vi "IVI DC Power Supply Main Page.vi"(8 "error in (no error)":errorcluster, 11 "Node Ptr":T1 format="%.0x") -> (0 "error out":errorcluster)   [LabVIEW 2011, in "IVI DC Power Supply Custom Device.lvlib"]
uses:
  IVI DC Power Supply Custom Device.lvlib
  <vilib>/NI Veristand/Custom Device API/Custom Device Item Ref.ctl
  Global.vi
  <vilib>/NI Veristand/Custom Device API/Get Item Property (String).vi
  <vilib>/NI Veristand/Custom Device API/Get Item Property (Double).vi
  <vilib>/NI Veristand/Custom Device API/Set Item Property (String).vi
  <vilib>/NI Veristand/Custom Device API/Set Item Property (Double).vi
  <vilib>/NI Veristand/Custom Device API/Custom Device API.lvlib
panel:
  in  "Desired Loop Rate (Hz)":dbl=0.5
  in  "Logical Name in MAX":string
  in  "Header":cluster{"Section Name":string}={"Section Name"="IVI DC Power Supply Settings"}
  in  "Description":string
  in  "IVI DC Power Supply Name":string
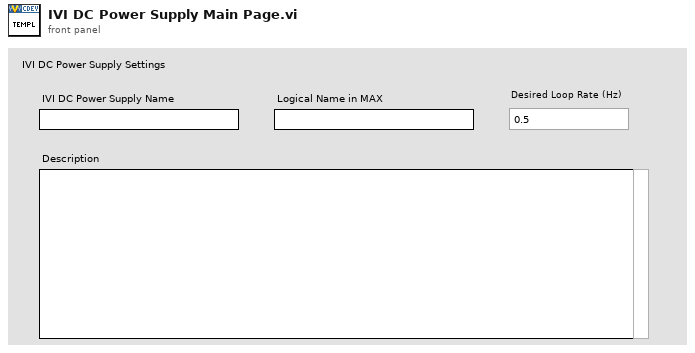
[diagram p1: front panel]
types:
  T1 = typedef "Custom Device API.lvlib/Custom Device Item Ref.ctl" = u64
  T2 = typedef "Custom Device API.lvlib/Custom Device Item Info.ctl" = cluster{"Name":string, "Is Channel":bool, "GUID":string}
  T3 = typedef "Custom Device API.lvlib/Custom Device Commands.ctl" = enum16{"Default", "Item renamed", "Shutdown", "Dynamic button pressed"}
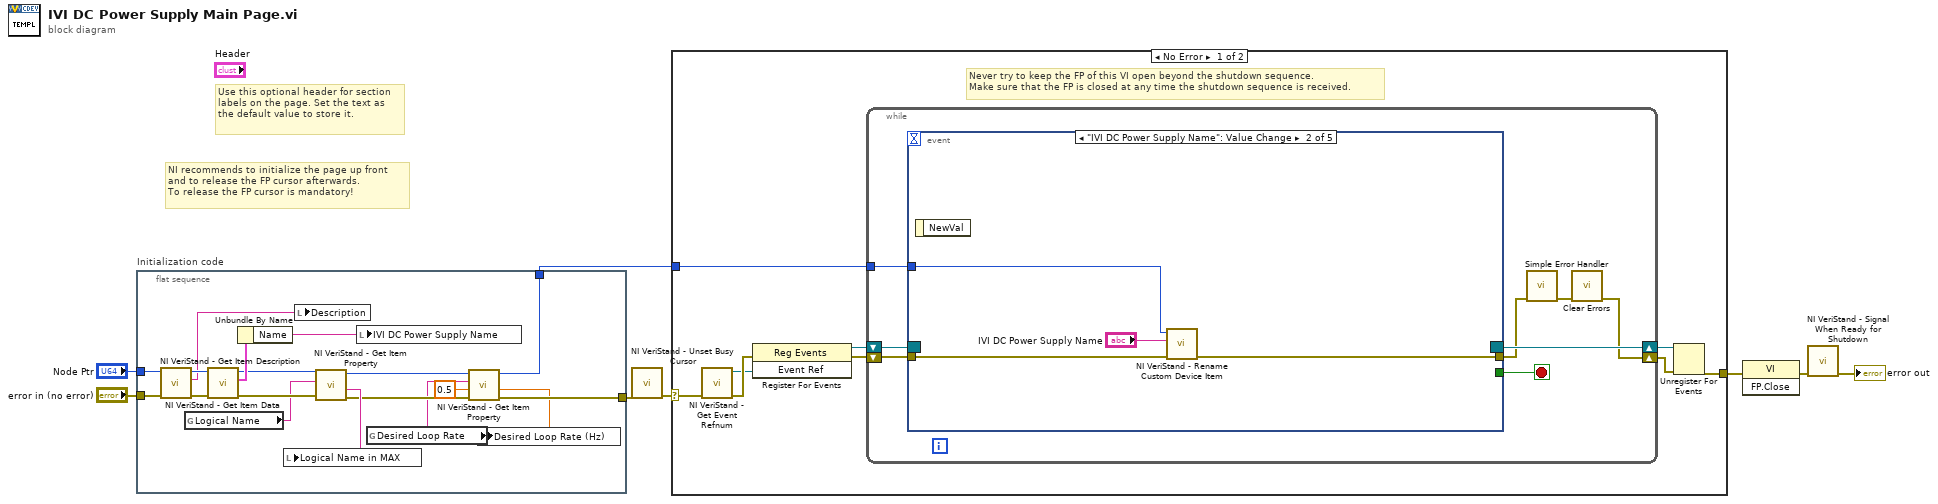
[diagram p0: block diagram]
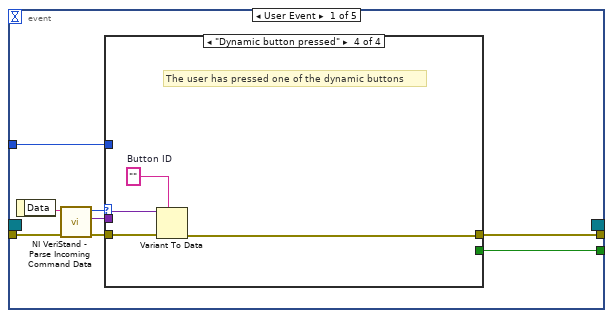
[diagram p2: hidden frame]
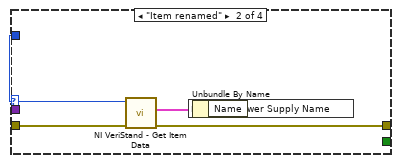
[diagram p4: hidden frame]
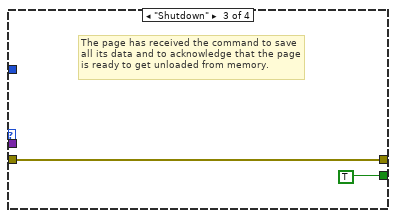
[diagram p5: hidden frame]
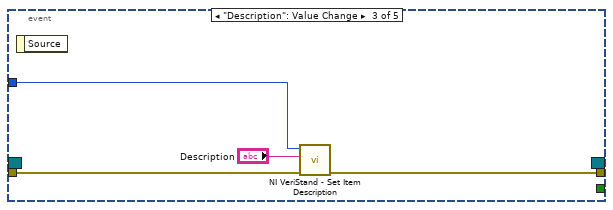
[diagram p6: hidden frame]
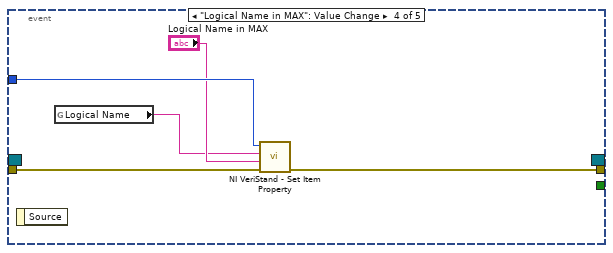
[diagram p7: hidden frame]
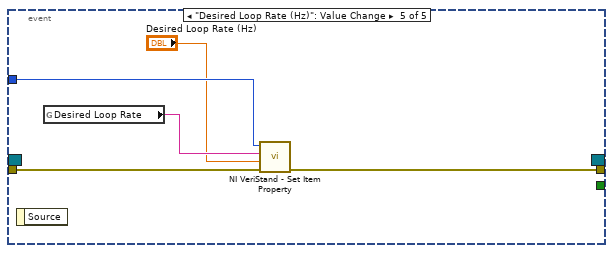
[diagram p8: hidden frame]
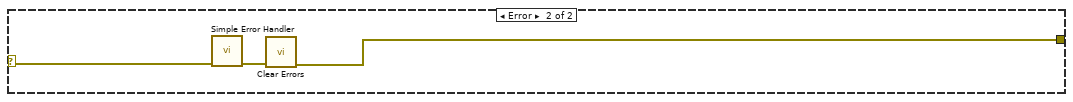
[diagram p9: hidden frame]
diagram:
  # "Use this optional header for section labels on the page. Set the text as the default value to store it."
  # "NI recommends to initialize the page up front\nand to release the FP cursor afterwards.\nTo release the FP cursor is mandatory!"
  n1 = flat-sequence "Initialization code" {
    tunnel: "error in (no error)" -> [w25]
    tunnel: "Node Ptr" -> [w24]
    tunnel: [w13] -> w2
    tunnel: [w12] -> w1
    frame #0 {
      n2 = call <vilib>:"NI VeriStand - Get Item Description.vi"("error in (no error)"=w25, "Item Ref in"=w24) -> ("error out"=w22:errorcluster, "Description"=w23:string, "Item Ref out"=w26:T1)  [unwired: 7 out]
      n3 = global read "Global.vi" "Logical Name"() -> (w17:string)
      n4 = call <vilib>:"NI VeriStand - Get Item Data.vi"("error in (no error)"=w22, "Item Ref in"=w26) -> ("error out"=w18:errorcluster, "Item Info"=w21:T2, "Item Ref out"=w19:T1)  [unwired: 7 out]
      n5 = Unbundle By Name(w21) -> ("Name"=w20:string)
      n6 = local write "Description"(w23) -> ()
      n7 = call-poly <vilib>:"NI VeriStand - Get Item Property.vi"("error in (no error)"=w18, "Property Name"=w17, "Item Ref in"=w19) -> ("error out"=w15:errorcluster, "Value"=w16:string, "Item Ref out"=w14:T1)  [unwired: 5 in, 1 out]
      n8 = local write "Logical Name in MAX"(w16) -> ()
      n9 = local write "IVI DC Power Supply Name"(w20) -> ()
      n10 = global read "Global.vi" "Desired Loop Rate"() -> (w11:string)
      n11 = call-poly <vilib>:"NI VeriStand - Get Item Property.vi"("error in (no error)"=w15, "Default Value"=0.5, "Property Name"=w11, "Item Ref in"=w14) -> ("error out"=w12:errorcluster, "Value"=w10:dbl, "Item Ref out"=w13:T1)  [unwired: 4 in, 1 out]
      n12 = local write "Desired Loop Rate (Hz)"(w10) -> ()
    }
  }
  n13 = call <vilib>:"NI VeriStand - Unset Busy Cursor.vi"("error in (no error)"=w1) -> ("error out"=w4:errorcluster)  [unwired: 10 out]
  n14 = case shown="No Error" w4 {
    selector: w4 -> [w27 w84]
    tunnel: [w32 w82] -> w8
    tunnel: w2 -> [w28 _]
    frame No Error {
      # "Never try to keep the FP of this VI open beyond the shutdown sequence.\nMake sure that the FP is closed at any time the shutdown sequence is received."
      n15 = call <vilib>:"NI VeriStand - Get Event Refnum.vi"("error in (no error)"=w27) -> ("error out"=w35:errorcluster, "Event Ref"=w31:refnum<user-event>)  [unwired: 9 out]
      n16 = register-events(error in=w35, w31) -> (reference out=w29:refnum<event-registration>, error out=w30:errorcluster)  [unwired: 1 in]
      n17 = while {
        tunnel: w28 -> [w39]
        shift-right: [w36] -> w33
        shift-left: w30 -> [w42]
        shift-right: [w43] -> w34
        shift-left: w29 -> [w41]
        stop <- w40 stop-if-true
        n18 = event shown="[1] \"IVI DC Power Supply Name\": Value Change" {
          selector: w41 -> [_ _ _ _ _]
          dyn-events: [_ _ _ _ _] -> w43
          timeout: _ -> [_ _ _ _ _]
          tunnel: w42 -> [w51 w67 w70 w76 w81]
          tunnel: [w47 _ _ _ _] -> w40
          tunnel: [w46 w66 w69 w75 w80] -> w38
          tunnel: w39 -> [w45 w65 w71 w74 w79]
          event User Event {
            n19 = event-data() -> ("Data"=w50:string)  [unwired: 1 out]
            n20 = call <vilib>:"NI VeriStand - Parse Incoming Command Data.vi"("error in (no error)"=w51, "Incoming data"=w50) -> ("error out"=w49:errorcluster, "Outgoing data"=w44:variant, "Action"=w48:T3)  [unwired: 7 out]
            n21 = case shown="\"Dynamic button pressed\"" w48 {
              tunnel: w49 -> [w52 w57 w58 w63]
              tunnel: [_ _ TRUE _] -> w47
              tunnel: [w52 w54 w58 w60] -> w46
              tunnel: w45 -> [_ w56 _ _]
              tunnel: w44 -> [_ _ _ w62]
              frame "Default", Default {
              }
              frame "Item renamed" {
                n22 = call <vilib>:"NI VeriStand - Get Item Data.vi"("error in (no error)"=w57, "Item Ref in"=w56) -> ("error out"=w54:errorcluster, "Item Info"=w55:T2)  [unwired: 8 out]
                n23 = Unbundle By Name(w55) -> ("Name"=w53:string)
                n24 = local write "IVI DC Power Supply Name"(w53) -> ()
              }
              frame "Shutdown" {
                # "The page has received the command to save all its data and to acknowledge that the page is ready to get unloaded from memory."
              }
              frame "Dynamic button pressed" {
                w61 = ""  # Button ID
                # "The user has pressed one of the dynamic buttons"
                n25 = Variant To Data(error in=w63, type=w61, Variant=w62) -> (error out=w60:errorcluster)  [unwired: 1 out]
              }
            }
          }
          event "IVI DC Power Supply Name": Value Change {
            n26 = event-data() -> ()  [unwired: 2 out]
            n27 = call <vilib>:"NI VeriStand - Rename Custom Device Item.vi"("error in (no error)"=w67, "New Name"="IVI DC Power Supply Name", "Item Ref in"=w65) -> ("error out"=w66:errorcluster)  [unwired: 8 out]
          }
          event "Description": Value Change {
            n28 = event-data() -> ()  [unwired: 2 out]
            n29 = call <vilib>:"NI VeriStand - Set Item Description.vi"("error in (no error)"=w70, "Description"="Description", "Item Ref in"=w71) -> ("error out"=w69:errorcluster)  [unwired: 8 out]
          }
          event "Logical Name in MAX": Value Change {
            n30 = event-data() -> ()  [unwired: 2 out]
            n31 = global read "Global.vi" "Logical Name"() -> (w72:string)
            n32 = call-poly <vilib>:"NI VeriStand - Set Item Property.vi"("error in (no error)"=w76, "Value"="Logical Name in MAX", "Property Name"=w72, "Item Ref in"=w74) -> ("error out"=w75:errorcluster)  [unwired: 5 in, 2 out]
          }
          event "Desired Loop Rate (Hz)": Value Change {
            n33 = event-data() -> ()  [unwired: 2 out]
            n34 = global read "Global.vi" "Desired Loop Rate"() -> (w78:string)
            n35 = call-poly <vilib>:"NI VeriStand - Set Item Property.vi"("error in (no error)"=w81, "Value"="Desired Loop Rate (Hz)", "Property Name"=w78, "Item Ref in"=w79) -> ("error out"=w80:errorcluster)  [unwired: 5 in, 2 out]
          }
        }
        n36 = call <vilib>:"Simple Error Handler.vi"("error in (no error)"=w38) -> ("error out"=w37:errorcluster)  [unwired: 1 in, 7 out]
        n37 = call <vilib>:"Clear Errors.vi"("error in (no error)"=w37) -> ("error out"=w36:errorcluster)  [unwired: 6 out]
      }
      n38 = Unregister For Events(event registration refnum=w34, error in=w33) -> (error out=w32:errorcluster)
    }
    frame Error {
      n39 = call <vilib>:"Simple Error Handler.vi"("error in (no error)"=w84) -> ("error out"=w83:errorcluster)  [unwired: 1 in, 7 out]
      n40 = call <vilib>:"Clear Errors.vi"("error in (no error)"=w83) -> ("error out"=w82:errorcluster)  [unwired: 6 out]
    }
  }
  n41 = invoke class="VI" method="FP.Close"(error in=w8) -> (error out=w7:errorcluster)  [unwired: 2 in, 2 out]
  n42 = call <vilib>:"NI VeriStand - Signal When Ready for Shutdown.vi"("error in (no error)"=w7) -> ("error out"=→"error out":errorcluster)  [unwired: 10 out]
